vi "Configure Standard Waveform(Harmonic).vi"(0 "VISA resource name":refnum<visa-resource-name>, 1 "Frequency (1000 Hz)":dbl=1000.0, 2 "Phase (0 Degree)":dbl, 5 "Output Channel (1: Channel 1)":i32(ring)=1 items=["Channel 1"=1, "Channel 2"=2], 7 "Amplitude (5 Vpp)":dbl=5.0, 9 "Amplitude Unit (0: Vpp)":i32(ring) items=["Vpp", "Vrms", "dBm"], 11 "error in (no error)":errorcluster, 12 "Offset (0)":dbl) -> (4 "VISA resource name out":refnum<visa-resource-name>, 15 "error out":errorcluster)   [LabVIEW 2012, in "RIGOL DG4000 Series.lvlib"]
doc: "Outputs a harmonic with specified frequency, amplitude, DC offset and start phase."
uses:
  <instrlib>/RIGOL DG4000 Series/RIGOL DG4000 Series.lvlib
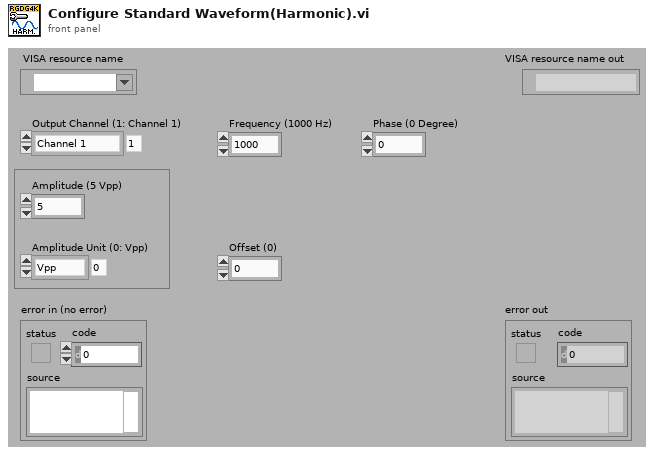
[diagram p1: front panel]
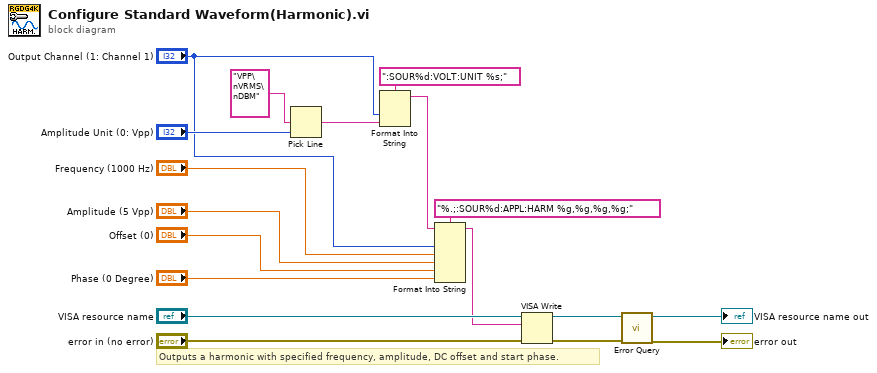
[diagram p0: block diagram]
diagram:
  # "Outputs a harmonic with specified frequency, amplitude, DC offset and start phase."
  n1 = Pick Line(multi-line string="VPP\nVRMS\nDBM", line index="Amplitude Unit (0: Vpp)") -> (output string=w10:string)  [unwired: 1 out]
  n2 = Format Into String(format string=":SOUR%d:VOLT:UNIT %s;", "Output Channel (1: Channel 1)", w10) -> (resulting string=w2:string)  [unwired: 2 in, 1 out]
  n3 = Format Into String(format string="%.;:SOUR%d:APPL:HARM %g,%g,%g,%g;", initial string=w2, "Output Channel (1: Channel 1)", "Frequency (1000 Hz)", "Amplitude (5 Vpp)", "Offset (0)", "Phase (0 Degree)") -> (resulting string=w1:string)  [unwired: 1 in, 1 out]
  n4 = VISA Write(VISA resource name="VISA resource name", write buffer=w1, error in (no error)="error in (no error)") -> (VISA resource name out=w7:refnum<visa-resource-name>, error out=w6:errorcluster)  [unwired: 1 out]
  n5 = call <instrlib>:"Error Query.vi"("error in (no error)"=w6, "VISA resource name"=w7) -> ("error out"=→"error out":errorcluster, "VISA resource name out"=→"VISA resource name out":refnum<visa-resource-name>)  [unwired: 8 out]
